vi "subtract.vi"(8 "error in (no error)":errorcluster, 11 "params":variant) -> (0 "error out":errorcluster, 3 "data":variant)   [LabVIEW 2017]
uses:
  <vilib>/National Instruments/Variant Data Manipulation/Path API/Read Value at Path(String).vi
  <vilib>/Utility/Data Type/NI_Data Type.lvlib
  <vilib>/National Instruments/Variant Data Manipulation/Variant Data Manipulation.lvlib
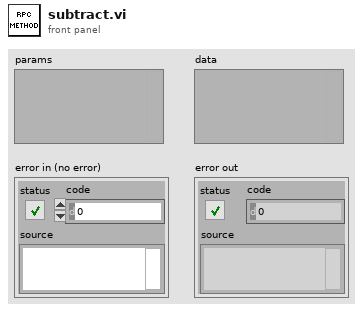
[diagram p1: front panel]
types:
  T1 = typedef "NI_Data Type.lvlib/Data Type.ctl" = enum8{"Invalid Type", "Void", "I8", "I16", "I32", "I64", "U8", "U16", "U32", "U64", "Single Float", "Double Float", "Extended Float", "Single Complex", "Double Complex", "Extended Complex", "Enum U8", "Enum U16", "Enum U32", "Enum U64", "Single Float With Unit", "Double Float With Unit", "Extended Float With Unit", "Single Complex with Unit", "Double Complex with Unit", "Extended Complex with Unit", "Boolean", "String", "Path", "Picture", "Tag", "Array", "Cluster", "Variant", "LV Variant", "Waveform", "Timestamp", "Digital Waveform", "Digital Data", "ExpressData", "Refnum", "External Data", "VI", "Poly VI", "LabVIEW Class Instance", "Fixed Point"}
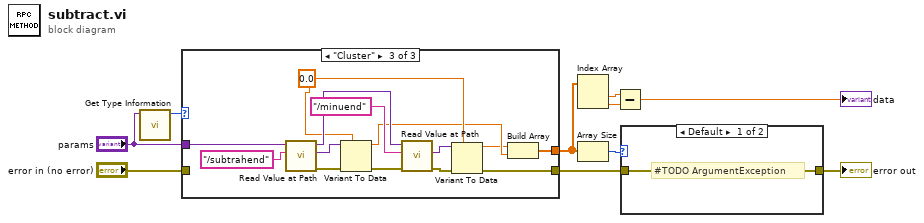
[diagram p0: block diagram]
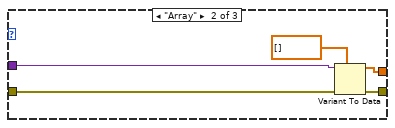
[diagram p4: hidden frame]
diagram:
  n1 = call <vilib>:"Get Type Information.vi"("Variant"="params") -> ("Type"=w9:T1)  [unwired: 6 in, 4 out]
  n2 = case shown="\"Cluster\"" w9 {
    tunnel: "error in (no error)" -> [w11 w16 _]
    tunnel: "params" -> [_ w15 w30]
    tunnel: [w11 w14 w21] -> w1
    tunnel: [_ w12 w17] -> w4
    frame Default {
      # "#TODO ArgumentException"
    }
    frame "Array" {
      n3 = Variant To Data(error in=w16, type=dbl[] [] ("x"), Variant=w15) -> (data=w12:dbl[], error out=w14:errorcluster)
    }
    frame "Cluster" {
      w20 = 0.0 ("double precision float")
      n4 = call-poly <vilib>:"Read Value at Path.vi"("Path String"="/subtrahend", "Variant in"=w30) -> ("error out"=w24:errorcluster, "Element out"=w25:variant, "Variant out"=w28:variant)  [unwired: 7 in]
      n5 = Variant To Data(error in=w24, type=w20, Variant=w25) -> (data=w19:dbl, error out=w23:errorcluster)
      n6 = call-poly <vilib>:"Read Value at Path.vi"("error in (no error)"=w23, "Path String"="/minuend", "Variant in"=w28) -> ("error out"=w22:errorcluster, "Element out"=w26:variant)  [unwired: 6 in, 1 out]
      n7 = Variant To Data(error in=w22, type=w20, Variant=w26) -> (data=w18:dbl, error out=w21:errorcluster)
      n8 = Build Array(w18, w19) -> (w17:dbl[])
    }
  }
  n9 = Index Array(array=w4) -> (element #1=w6:dbl, element #2=w5:dbl)  [unwired: 2 in]
  n10 = Array Size(array=w4) -> (size(s)=w3:i32)
  n11 = Subtract(x=w6, y=w5) -> (x-y=→"data":dbl)
  n12 = case shown="Default" w3 {
    tunnel: [w31 w32] -> w2
    tunnel: w1 -> [w31 w32]
    frame Default {
      # "#TODO ArgumentException"
    }
    frame 2 {
    }
  }
  "error out" <- w2
